vi "主动发送数据生成Condition(子VI).vi"(7 "结束时间":timestamp, 8 "数据发送协议":enum16{"2005-212协议", "2017-212协议"}(ring)=enum."2017-212协议", 9 "database":string, 10 "Label.Text":string, 11 "数值":i32) -> (0 "date/time string":string, 1 "database溢出":bool, 2 "columns":string[](array[string])=["时间", "测量模式", "数据类型", "检测值", "单位", "数据标识"], 3 "CONDITION":string)   [LabVIEW 2016, in "数据传输系统.lvlib"]
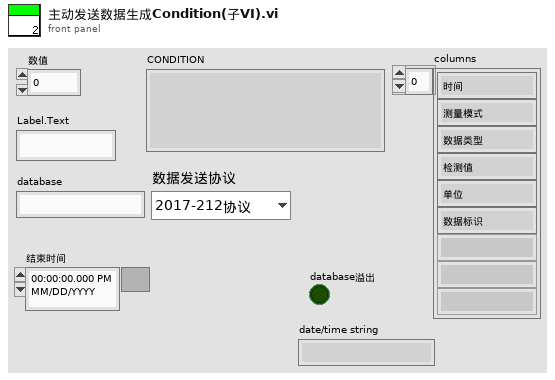
[diagram p1: front panel]
types:
  T1 = cluster{"time1":string, "time2":string, "time3":string, "time4":string, "time5":string, "time6":string, "time7":string, "time8":string, "time9":string, "time10":string, "time11":string, "time12":string, "time13":string, "time14":string, "time15":string, "time16":string, "time17":string, "time18":string, "time19":string, "time20":string, "time21":string, "time22":string, "time23":string, "time24":string, "time25":string, "time26":string, "time27":string, "time28":string, "time29":string, "time30":string, "time31":string, "time32":string, "time33":string, "time34":string, "time35":string, "time36":string, "time37":string, "time38":string}
  T2 = typedef "LVDateTimeRec.ctl" = cluster{"秒数的小数部分":dbl, "秒":i32, "分":i32, "时":i32, "日":i32, "月":i32, "年":i32, "天数（周）":i32, "天数（年）":i32, "DST":i32}
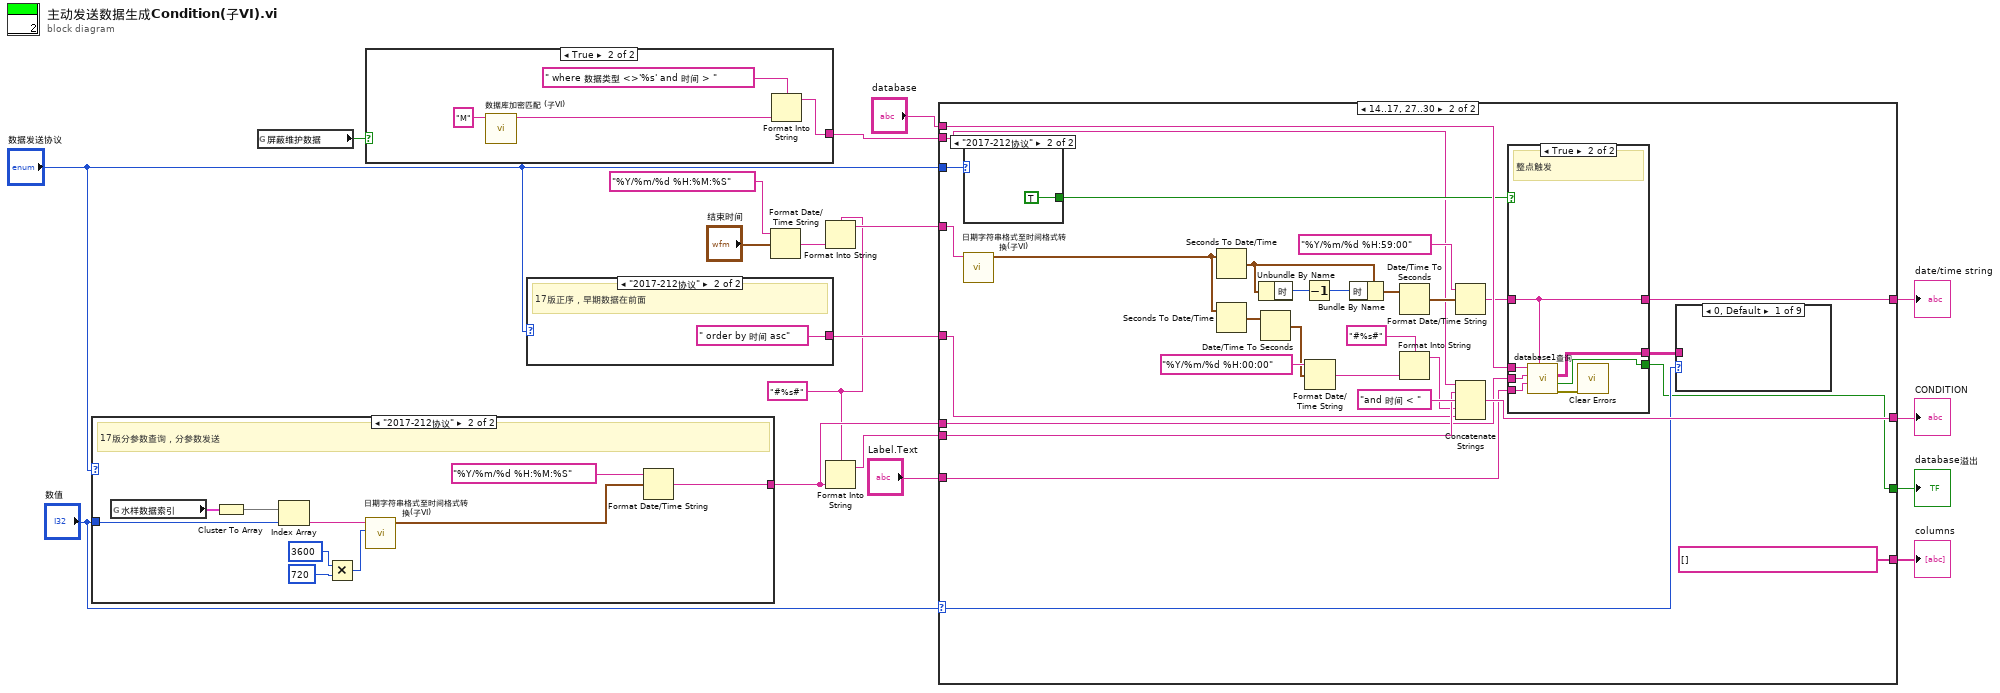
[diagram p0: block diagram]
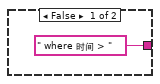
[diagram p2: hidden frame]
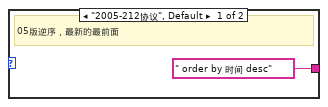
[diagram p3: hidden frame]
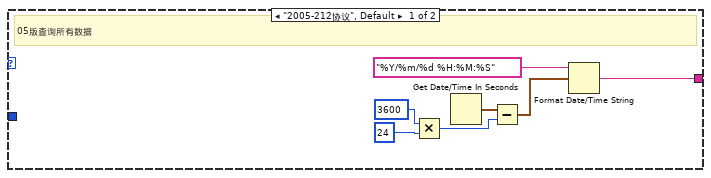
[diagram p4: hidden frame]
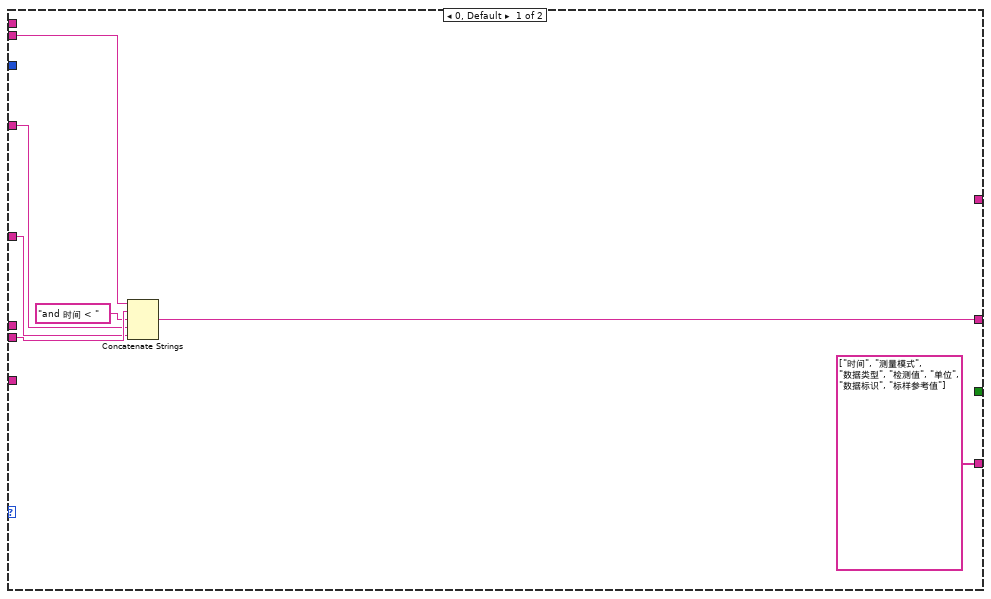
[diagram p5: hidden frame]
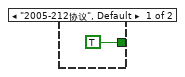
[diagram p6: hidden frame]
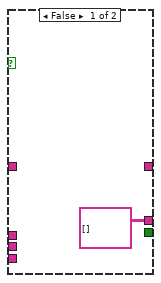
[diagram p7: hidden frame]
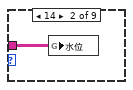
[diagram p8: hidden frame]
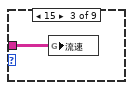
[diagram p9: hidden frame]
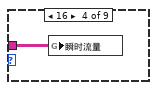
[diagram p10: hidden frame]
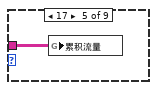
[diagram p11: hidden frame]
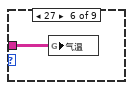
[diagram p12: hidden frame]
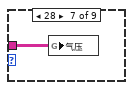
[diagram p13: hidden frame]
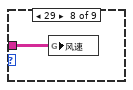
[diagram p14: hidden frame]
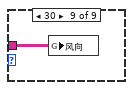
[diagram p15: hidden frame]
diagram:
  w6 = "#%s#" ("初始字符串")
  n1 = case shown="\"2017-212协议\"" "数据发送协议" {
    tunnel: [w24 w27] -> w18
    tunnel: "数值" -> [_ w33]
    frame "2005-212协议", Default {
      # "05版查询所有数据"
      n2 = Multiply(x=3600, y=24) -> (x*y=w19:i32)
      n3 = Get Date/Time In Seconds() -> (seconds since 1Jan1904=w23:timestamp)
      n4 = Subtract(x=w23, y=w19) -> (x-y=w22:timestamp)
      n5 = Format Date/Time String(time format string (%c)="%Y/%m/%d %H:%M:%S" ("时间格式字符串(%c)"), seconds (now)=w22) -> (date/time string=w24:string)  [unwired: 1 in]
    }
    frame "2017-212协议" {
      # "17版分参数查询，分参数发送"
      n6 = global read "全局 水样时间.vi" "水样数据索引"() -> (w34:T1)
      n7 = Cluster To Array(cluster=w34) -> (array=w35:string[])
      n8 = Index Array(array=w35, index=w33) -> (element=w32:string)
      n9 = Multiply(x=3600, y=720) -> (x*y=w29:i32)
      n10 = call "日期字符串格式至时间格式转换(子VI).vi"("数值"=w29, "data[0]"=w32) -> ("time stamp"=w26:timestamp)  [unwired: 9 in]
      n11 = Format Date/Time String(time format string (%c)="%Y/%m/%d %H:%M:%S" ("时间格式字符串(%c)"), seconds (now)=w26) -> (date/time string=w27:string)  [unwired: 1 in]
    }
  }
  n12 = global read "断电保存全局.vi" "屏蔽维护数据"() -> (w4:bool)
  n13 = case shown="True" w4 {
    tunnel: [" where 时间 > " w39] -> w5
    frame False {
    }
    frame True {
      n14 = call "数据库加密匹配 (子VI).vi"("输入参数"="M") -> ("Encoded String"=w37:string)  [unwired: 10 in]
      n15 = Format Into String(format string=" where 数据类型 <>'%s' and 时间 > ", w37) -> (resulting string=w39:string)  [unwired: 2 in, 1 out]
    }
  }
  n16 = case shown="\"2017-212协议\"" "数据发送协议" {
    tunnel: [" order by 时间 desc" ("字符串") " order by 时间 asc" ("字符串")] -> w12
    frame "2005-212协议", Default {
      # "05版逆序，最新的最前面"
    }
    frame "2017-212协议" {
      # "17版正序，早期数据在前面"
    }
  }
  n17 = Format Date/Time String(time format string (%c)="%Y/%m/%d %H:%M:%S" ("时间格式字符串(%c)"), seconds (now)="结束时间") -> (date/time string=w3:string)  [unwired: 1 in]
  n18 = Format Into String(format string=w6, w3) -> (resulting string=w14:string)  [unwired: 2 in, 1 out]
  n19 = Format Into String(format string=w6, w18) -> (resulting string=w13:string)  [unwired: 2 in, 1 out]
  n20 = case shown="14..17, 27..30" "数值" {
    selector: "数值" -> [_ w73]
    tunnel: w13 -> [w49 w77]
    tunnel: [w48 w78] -> w8
    tunnel: w14 -> [w46 w50]
    tunnel: "database" -> [_ w76]
    tunnel: "Label.Text" -> [_ w75]
    tunnel: w18 -> [_ w61]
    tunnel: w12 -> [w45 w72]
    tunnel: [string[] ["时间", "测量模式", "数据类型", "检测值", "单位", "数据标识", "标样参考值"] ("columns") string[] [] ("columns")] -> w11
    tunnel: "数据发送协议" -> [_ w69]
    tunnel: w5 -> [w43 w60]
    tunnel: [_ w52] -> w1
    tunnel: [_ w51] -> w2
    frame 0, Default {
      n21 = Concatenate Strings(w43, w49, "and 时间 < " ("字符串"), w46, w45) -> (w48:string)
    }
    frame 14..17, 27..30 {
      n22 = case shown="\"2017-212协议\"" w69 {
        tunnel: [TRUE TRUE] -> w71
        frame "2005-212协议", Default {
        }
        frame "2017-212协议" {
        }
      }
      n23 = call "日期字符串格式至时间格式转换(子VI).vi"("data[0]"=w50) -> ("time stamp"=w57:timestamp)  [unwired: 10 in]
      n24 = Seconds To Date/Time(time stamp (now)=w57) -> (date time rec=w66:T2)  [unwired: 1 in]
      n25 = Seconds To Date/Time(time stamp (now)=w57) -> (date time rec=w56:T2)  [unwired: 1 in]
      n26 = Unbundle By Name(w66) -> ("时"=w67:i32)
      n27 = Date/Time To Seconds(2:w56) -> (0:w58:timestamp)  [unwired: 1 in]
      n28 = Decrement(x=w67) -> (x-1=w68:i32)
      n29 = Format Date/Time String(time format string (%c)="%Y/%m/%d %H:00:00" ("时间格式字符串(%c)"), seconds (now)=w58) -> (date/time string=w54:string)  [unwired: 1 in]
      n30 = Bundle By Name(cluster=w66, "时"=w68) -> (w65:T2)
      n31 = Date/Time To Seconds(2:w65) -> (0:w64:timestamp)  [unwired: 1 in]
      n32 = Format Into String(format string="#%s#" ("初始字符串"), w54) -> (resulting string=w53:string)  [unwired: 2 in, 1 out]
      n33 = Format Date/Time String(time format string (%c)="%Y/%m/%d %H:59:00" ("时间格式字符串(%c)"), seconds (now)=w64) -> (date/time string=w62:string)  [unwired: 1 in]
      n34 = Concatenate Strings(w60, w77, "and 时间 < " ("字符串"), w53, w72) -> (w78:string)
      n35 = case shown="True" w71 {
        tunnel: w76 -> [_ w89]
        tunnel: w75 -> [_ w88]
        tunnel: [string[][] [] ("data") w87] -> w74
        tunnel: w62 -> [_ w84]
        tunnel: w61 -> [_ w85]
        tunnel: [_ w84] -> w52
        tunnel: [_ w83] -> w51
        frame False {
        }
        frame True {
          # "整点触发"
          n36 = call "database1查询.vi"("时间2"=w84, "table"=w88, "时间1"=w85, "database"=w89) -> ("error out"=w86:errorcluster, "database溢出"=w83:bool, "data"=w87:string[][])  [unwired: 3 in, 1 out]
          n37 = call <vilib>:"Clear Errors.vi"("error in (no error)"=w86) -> ()  [unwired: 5 in, 2 out]
        }
      }
      n38 = case shown="0, Default" w73 {
        tunnel: w74 -> [_ w90 w91 w92 w93 w94 w95 w96 w97]
        frame 0, Default {
        }
        frame 14 {
          n39 = global write "全局 所有参数.vi" "水位"(w90) -> ()
        }
        frame 15 {
          n40 = global write "全局 所有参数.vi" "流速"(w91) -> ()
        }
        frame 16 {
          n41 = global write "全局 所有参数.vi" "瞬时流量"(w92) -> ()
        }
        frame 17 {
          n42 = global write "全局 所有参数.vi" "累积流量"(w93) -> ()
        }
        frame 27 {
          n43 = global write "全局 所有参数.vi" "气温"(w94) -> ()
        }
        frame 28 {
          n44 = global write "全局 所有参数.vi" "气压"(w95) -> ()
        }
        frame 29 {
          n45 = global write "全局 所有参数.vi" "风速"(w96) -> ()
        }
        frame 30 {
          n46 = global write "全局 所有参数.vi" "风向"(w97) -> ()
        }
      }
    }
  }
  "CONDITION" <- w8
  "columns" <- w11
  "database溢出" <- w2
  "date/time string" <- w1
